vi "Open.vi"(8 "error in (no error)":errorcluster, 11 "ODBC-Interface in":refnum<class "ODBC-Interface.lvclass">) -> (0 "error out":errorcluster, 3 "ODBC-Interface out":refnum<class "ODBC-Interface.lvclass">)   [LabVIEW 2014, in "DB-Configuration.lvlib" / "ODBC-Interface.lvclass"]
doc: "Open connection to ODBC database."
uses:
  ODBC-Interface.lvclass
  ODBC-Interface.lvclass/ODBC-Interface.ctl
  <vilib>/addons/database/Connection.llb/DB Tools Open Connec (String).vi
  <vilib>/addons/database/NI_Database_API.lvlib
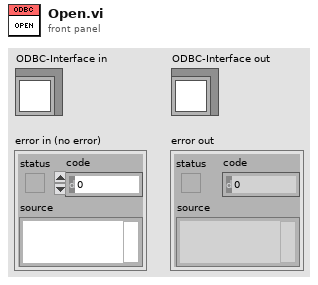
[diagram p1: front panel]
types:
  T1 = typedef "NI_Database_API.lvlib/Conn ObjectReference.ctl" = refnum<k1>
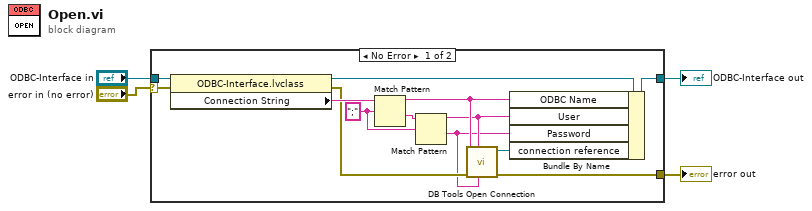
[diagram p0: block diagram]
diagram:
  n1 = case shown="No Error" "error in (no error)" {
    selector: "error in (no error)" -> [w6 w18]
    tunnel: "ODBC-Interface in" -> [w17 w19]
    tunnel: [w9 w18] -> w3
    tunnel: [w7 w19] -> w2
    frame No Error {
      w14 = ";" ("regular expression")
      n2 = property class="ODBC-Interface.lvclass"(reference=w17, error in=w6) -> (reference out=w8:refnum<class "ODBC-Interface.lvclass">, error out=w11:errorcluster, "Connection String"=w16:string)
      n3 = Match Pattern(string=w16, regular expression=w14) -> (before substring=w13:string, after substring=w15:string)  [unwired: 1 in, 2 out]
      n4 = Match Pattern(string=w15, regular expression=w14) -> (before substring=w12:string, after substring=w5:string)  [unwired: 1 in, 2 out]
      n5 = call-poly <vilib>:"DB Tools Open Connection.vi"("password"=w5, "userID"=w12, "error in (no error)"=w11, "connection information"=w13) -> ("error out"=w9:errorcluster, "connection reference"=w10:T1)  [unwired: 4 in]
      n6 = Bundle By Name(cluster=w8, "ODBC Name"=w13, "User"=w12, "Password"=w5, "connection reference"=w10) -> (w7:refnum<class "ODBC-Interface.lvclass">)
    }
    frame Error {
    }
  }
  "error out" <- w3
  "ODBC-Interface out" <- w2
